vi "scale-includer.vi"(2 "All Scale Notes":bool[][][](array[boolean]), 3 "Selected scales":bool[](array[boolean]), 4 "All Scale Names":string[][](array[string])) -> (0 "Selected Scale Notes":bool[][](array[boolean]), 1 "Selected Scale Names":string[](array[string]))   [LabVIEW 2019]
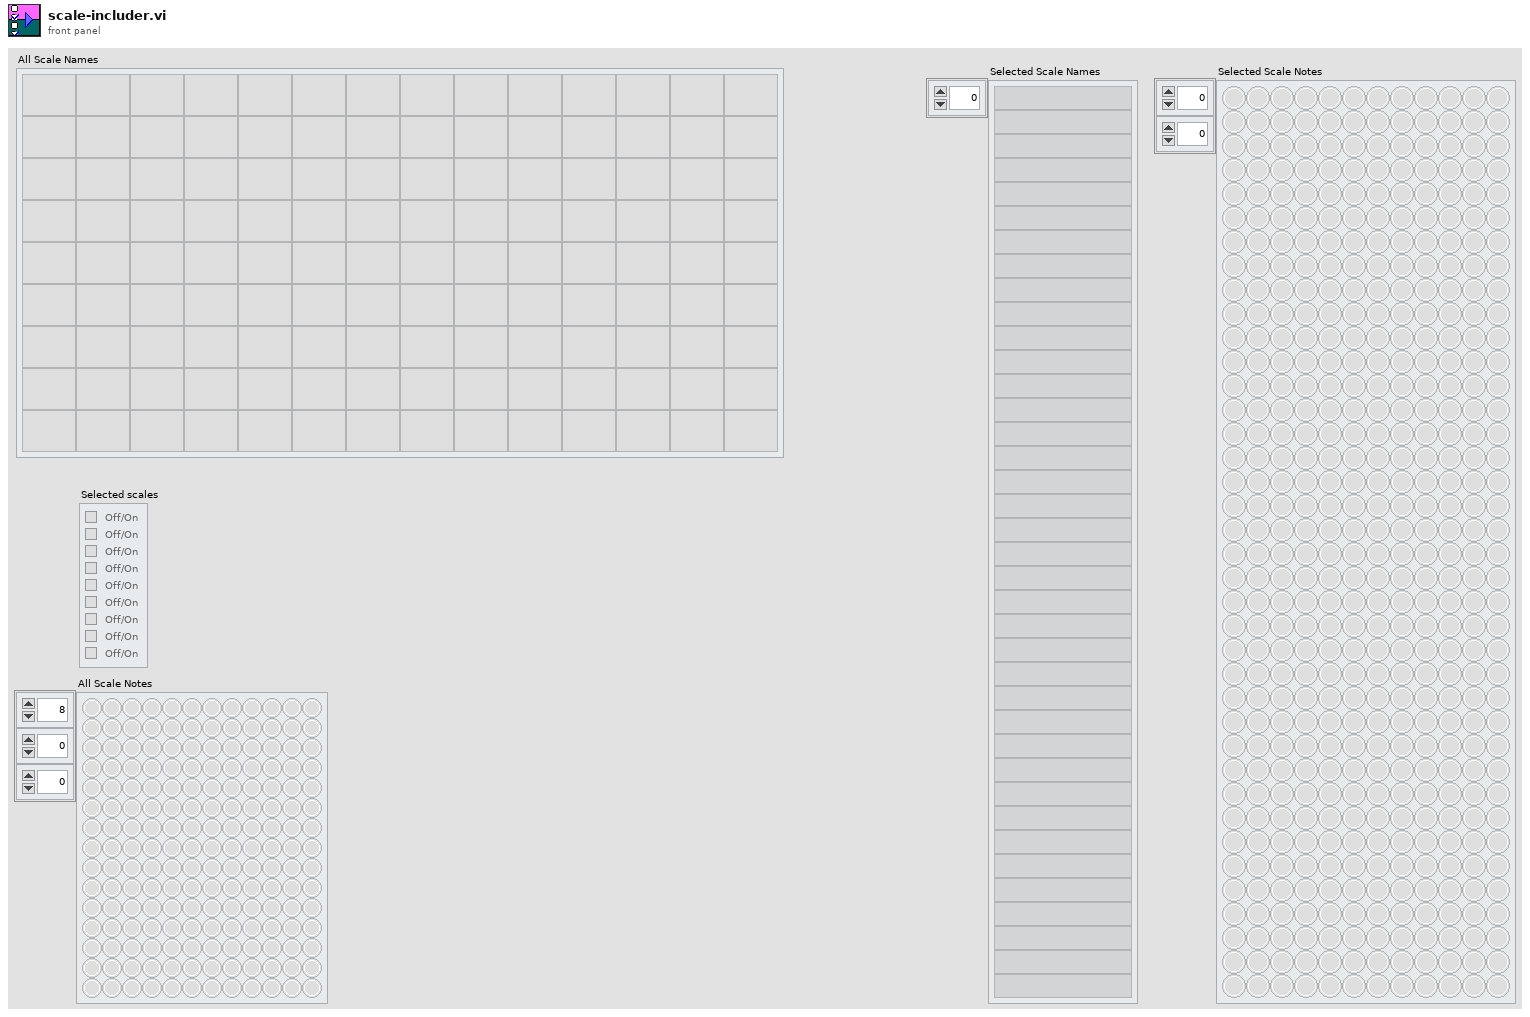
[diagram p1: front panel]
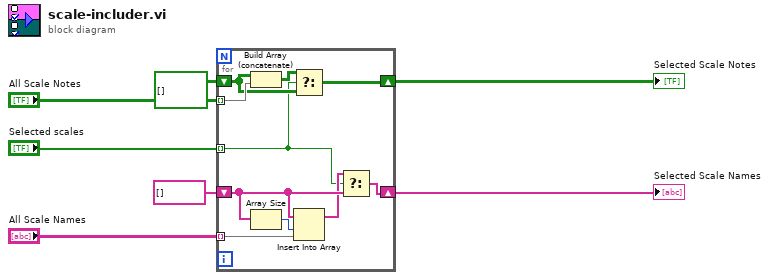
[diagram p0: block diagram]
diagram:
  n1 = for {
    tunnel: "All Scale Names" -> [w16] mode=indexing
    shift-right: [w17] -> w4
    shift-left: string[] [] -> [w15]
    shift-right: [w12] -> w6
    shift-left: bool[][] [] -> [w9]
    tunnel: "All Scale Notes" -> [w11] mode=indexing
    tunnel: "Selected scales" -> [w8] mode=indexing
    n2 = Build Array (concatenate)(w9, w11) -> (w10:bool[][])
    n3 = Array Size(array=w15) -> (size(s)=w14:i32)
    n4 = Select(t=w10, s=w8, f=w9) -> (s? t:f=w12:bool[][])
    n5 = Insert Into Array(array=w15, index=w14, new element=w16) -> (w13:string[])
    n6 = Select(t=w13, s=w8, f=w15) -> (s? t:f=w17:string[])
  }
  "Selected Scale Notes" <- w6
  "Selected Scale Names" <- w4
